vi "Generate.vi"(8 "error in (no error)":errorcluster, 10 "grpc-labview code gen path":path, 11 "grpc-labview generation params":T1={"Proto File Path"=[], "Import Paths"=[], "Prototype Library"=path "", "Target Project"=path "", "Target Name"="", "Generated Library Name"="", "Library Suffix"="", "Generate"=enum."Both"}) -> (0 "error out":errorcluster)   [LabVIEW 2020]
uses:
  grpc-labview Template Options.ctl
  044a0739-89e1-4b1a-922d-3cd0be8340d7.vi
  4f1e07c7-134f-48bf-9e2b-32168593eea6.vi
  b7ffc98f-c339-4f2b-be22-195df47554a0.vi
  91d97991-0b99-4e09-b432-08e3dce16f9b.vi
  b7ffc98f-c339-4f2b-be22-195df47554a0.vi/3adaac93-9b8c-409d-b0b6-3665bc9ad28b.vi
  91d97991-0b99-4e09-b432-08e3dce16f9b.vi/3adaac93-9b8c-409d-b0b6-3665bc9ad28b.vi
  Get Absolute Source Dir Path.vi
  <vilib>/Utility/Data Type/NI_Data Type.lvlib
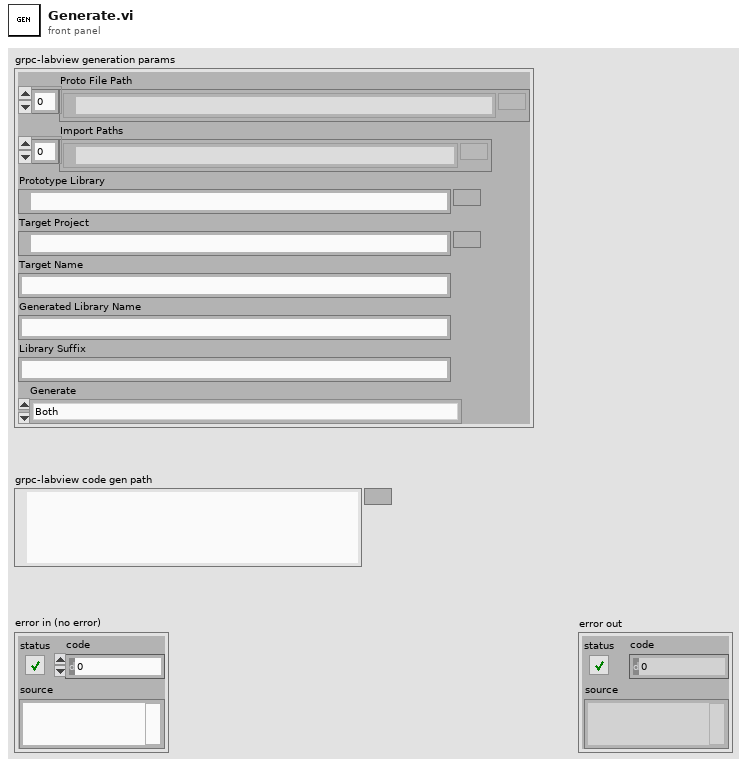
[diagram p1: front panel]
types:
  T1 = typedef "grpc-labview Template Options.ctl" = cluster{"Proto File Path":path[], "Import Paths":path[], "Prototype Library":path, "Target Project":path, "Target Name":string, "Generated Library Name":string, "Library Suffix":string, "Generate":enum16{"gRPC Server", "gRPC Client", "Both"}}
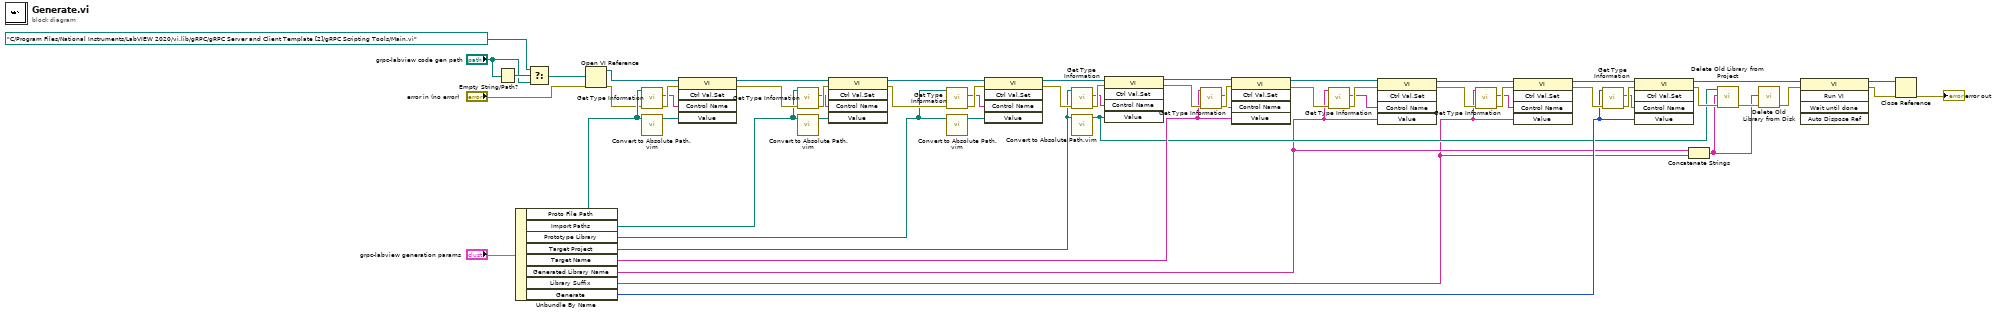
[diagram p0: block diagram]
diagram:
  n1 = Empty String/Path?(string/path="grpc-labview code gen path") -> (empty?=w45:bool)
  n2 = Unbundle By Name("grpc-labview generation params") -> ("Proto File Path"=w10:path[], "Import Paths"=w33:path[], "Prototype Library"=w29:path, "Target Project"=w9:path, "Target Name"=w21:string, "Generated Library Name"=w2:string, "Library Suffix"=w1:string, "Generate"=w11:enum16{"gRPC Server", "gRPC Client", "Both"})
  n3 = Select(t=path "C:/Program Files/National Instruments/LabVIEW 2020/vi.lib/gRPC/gRPC Server and Client Template [2]/gRPC Scripting Tools/Main.vi", s=w45, f="grpc-labview code gen path") -> (s? t:f=w42:path)
  n4 = Open VI Reference(vi path=w42, error in (no error)="error in (no error)") -> (vi reference=w58:refnum<vi>, error out=w8:errorcluster)  [unwired: 4 in]
  n5 = call <vilib>:"Get Type Information.vi"("error in (no error)"=w8, "variant"=w10) -> ("error out"=w38:errorcluster, "name"=w37:string)  [unwired: 5 in, 3 out]
  n6 = call "Convert to Absolute Path.vim"("relative path"=w10) -> ("absolute path"=w36:path[])  [unwired: 10 in]
  n7 = invoke class="VI" method="Ctrl Val.Set"(reference=w58, error in=w38, "Control Name"=w37, "Value"=w36) -> (reference out=w56:refnum<vi>, error out=w35:errorcluster)  [unwired: 1 in, 3 out]
  n8 = call <vilib>:"Get Type Information.vi"("error in (no error)"=w35, "variant"=w33) -> ("error out"=w34:errorcluster, "name"=w32:string)  [unwired: 5 in, 3 out]
  n9 = call "Convert to Absolute Path.vim"("relative path"=w33) -> ("absolute path"=w46:path[])  [unwired: 10 in]
  n10 = invoke class="VI" method="Ctrl Val.Set"(reference=w56, error in=w34, "Control Name"=w32, "Value"=w46) -> (reference out=w55:refnum<vi>, error out=w31:errorcluster)  [unwired: 1 in, 3 out]
  n11 = call <vilib>:"Get Type Information.vi"("error in (no error)"=w31, "variant"=w29) -> ("error out"=w30:errorcluster, "name"=w28:string)  [unwired: 5 in, 3 out]
  n12 = call "Convert to Absolute Path.vim"("relative path"=w29) -> ("absolute path"=w39:path)  [unwired: 10 in]
  n13 = invoke class="VI" method="Ctrl Val.Set"(reference=w55, error in=w30, "Control Name"=w28, "Value"=w39) -> (reference out=w54:refnum<vi>, error out=w27:errorcluster)  [unwired: 1 in, 3 out]
  n14 = call <vilib>:"Get Type Information.vi"("error in (no error)"=w27, "variant"=w9) -> ("error out"=w26:errorcluster, "name"=w25:string)  [unwired: 5 in, 3 out]
  n15 = call "Convert to Absolute Path.vim"("relative path"=w9) -> ("absolute path"=w4:path)  [unwired: 10 in]
  n16 = invoke class="VI" method="Ctrl Val.Set"(reference=w54, error in=w26, "Control Name"=w25, "Value"=w4) -> (reference out=w53:refnum<vi>, error out=w24:errorcluster)  [unwired: 1 in, 3 out]
  n17 = call <vilib>:"Get Type Information.vi"("error in (no error)"=w24, "variant"=w21) -> ("error out"=w23:errorcluster, "name"=w22:string)  [unwired: 5 in, 3 out]
  n18 = invoke class="VI" method="Ctrl Val.Set"(reference=w53, error in=w23, "Control Name"=w22, "Value"=w21) -> (reference out=w52:refnum<vi>, error out=w20:errorcluster)  [unwired: 1 in, 3 out]
  n19 = call <vilib>:"Get Type Information.vi"("error in (no error)"=w20, "variant"=w2) -> ("error out"=w19:errorcluster, "name"=w18:string)  [unwired: 5 in, 3 out]
  n20 = invoke class="VI" method="Ctrl Val.Set"(reference=w52, error in=w19, "Control Name"=w18, "Value"=w2) -> (reference out=w51:refnum<vi>, error out=w17:errorcluster)  [unwired: 1 in, 3 out]
  n21 = call <vilib>:"Get Type Information.vi"("error in (no error)"=w17, "variant"=w1) -> ("error out"=w16:errorcluster, "name"=w15:string)  [unwired: 5 in, 3 out]
  n22 = invoke class="VI" method="Ctrl Val.Set"(reference=w51, error in=w16, "Control Name"=w15, "Value"=w1) -> (reference out=w50:refnum<vi>, error out=w14:errorcluster)  [unwired: 1 in, 3 out]
  n23 = call <vilib>:"Get Type Information.vi"("error in (no error)"=w14, "variant"=w11) -> ("error out"=w13:errorcluster, "name"=w12:string)  [unwired: 5 in, 3 out]
  n24 = invoke class="VI" method="Ctrl Val.Set"(reference=w50, error in=w13, "Control Name"=w12, "Value"=w11) -> (reference out=w49:refnum<vi>, error out=w7:errorcluster)  [unwired: 1 in, 3 out]
  n25 = Concatenate Strings(w2, w1) -> (w3:string)
  n26 = call "Delete Old Library from Project.vi"("error in (no error)"=w7, "folder to delete"=w3, "path to project"=w4) -> ("error out"=w6:errorcluster)  [unwired: 8 in]
  n27 = call "Delete Old Library from Disk.vi"("error in (no error)"=w6, "folder to delete"=w3) -> ("error out"=w5:errorcluster)  [unwired: 9 in]
  n28 = invoke class="VI" method="Run VI"(reference=w49, error in=w5) -> (reference out=w48:refnum<vi>, error out=w47:errorcluster)  [unwired: 3 in, 3 out]
  n29 = Close Reference(reference=w48, error in (no error)=w47) -> (error out=→"error out":errorcluster)
